vi "STR_ASCII-Unicode.vi"(1 "ASCII string":string caption="ASCII字符串") -> (0 "unicode string":string caption="unicode字符串")   [LabVIEW 2012]
doc: "This VI converts an ASCII string to a unicode string."
uses:
  kernel32.dll
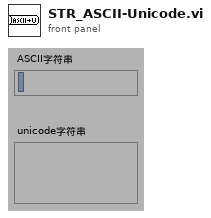
[diagram p1: front panel]
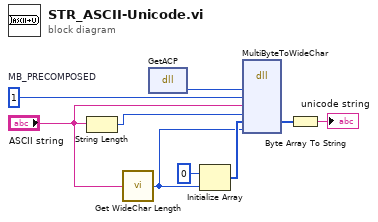
[diagram p0: block diagram]
diagram:
  w9 = u32 1  # MB_PRECOMPOSED
  n1 = String Length(string="ASCII string") -> (length=w6:i32)
  n2 = call "Get WideChar Length.vi"("ASCII string"="ASCII string") -> ("Byte Length"=w1:i32)
  n3 = dll-call lib="kernel32.dll" fn="GetACP" label="GetACP()"() -> (w5:u32)  [unwired: 3 in, 2 out]
  n4 = Initialize Array(u8 0 ("元素"), w1) -> (w2:u8[])
  n5 = dll-call lib="kernel32.dll" fn="MultiByteToWideChar"("codePage"=w5, "dwFlags"=w9, "lpCStr"="ASCII string", "nChars"=w6, "lpWStr"=w2, "nWStr"=w1) -> ("lpWStr"=w8:u8[])  [unwired: 8 in, 3 out]
  n6 = Byte Array To String(unsigned byte array=w8) -> (string=→"unicode string":string)
